vi "Velocity Converter- magnitude-heading  to dx-dy.vi"(10 "Magnitude":dbl, 11 "Heading":T1 format="%05.1f") -> (3 "Vector Out":T2 {"East" format="%#_5g"})   [LabVIEW 2011]
doc: "Converts velocity in the Direction/Speed format (as defined in the appropriate Typedef) to X/Y velocity, which is the standard type within our architecture."
uses:
  2 Typedefs/Velocity.ctl
  2 Typedefs/heading.ctl
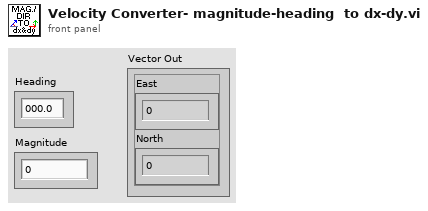
[diagram p1: front panel]
types:
  T1 = typedef "heading.ctl" = dbl
  T2 = typedef "Velocity.ctl" = cluster{"East":dbl, "North":dbl}
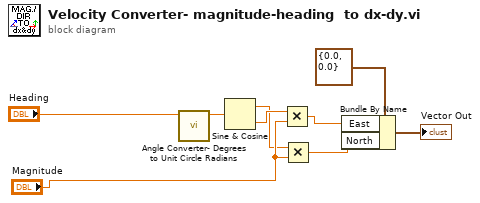
[diagram p0: block diagram]
diagram:
  n1 = call "Angle Converter- Degrees to Unit Circle Radians.vi"("Angle in \nHeading \nFormat"="Heading") -> ("Angle in \nUnit Circle\nRadians"=w4:dbl)  [unwired: 10 in]
  n2 = Sine & Cosine(0:w4) -> (1:w2:dbl, 2:w3:dbl)
  n3 = Multiply(x=w3, y="Magnitude") -> (x*y=w8:dbl)
  n4 = Multiply(x=w2, y="Magnitude") -> (x*y=w9:dbl)
  n5 = Bundle By Name(cluster=T2 {"East"=0.0, "North"=0.0} ("Velocity"), "East"=w8, "North"=w9) -> (→"Vector Out":T2)
